vi "Generate Doku Syntax.vi"(5 "GitHub Base Path":string="https://github.com/labviewhacker/LVH-Toolbox/raw/master/LabVIEW/vi.lib/LabVIEW%20Hacker/LVH-Toolbox/Common/Public/", 7 "Image Base Path":string="lib/exe/fetch.php?media=wiki:playground:dokugen:", 8 "Error In":errorcluster, 10 "VIs":T1[](array[typedef]), 11 "Doc Config":T2) -> (0 "Error Out":errorcluster)   [LabVIEW 2014, in "LMH-Toolbox.lvlib" / "LMH-Documentation.lvlib"]
uses:
  <vilib>/MakerHub/Toolbox/Private/Documentation/LMH-Documentation.lvlib
  <vilib>/MakerHub/Toolbox/Private/Documentation/Private/Type Defs/Doc Config.ctl
  <vilib>/MakerHub/Toolbox/Private/Documentation/Private/Type Defs/VI.ctl
panel:
  out "array of strings 2":string[][](array[string])
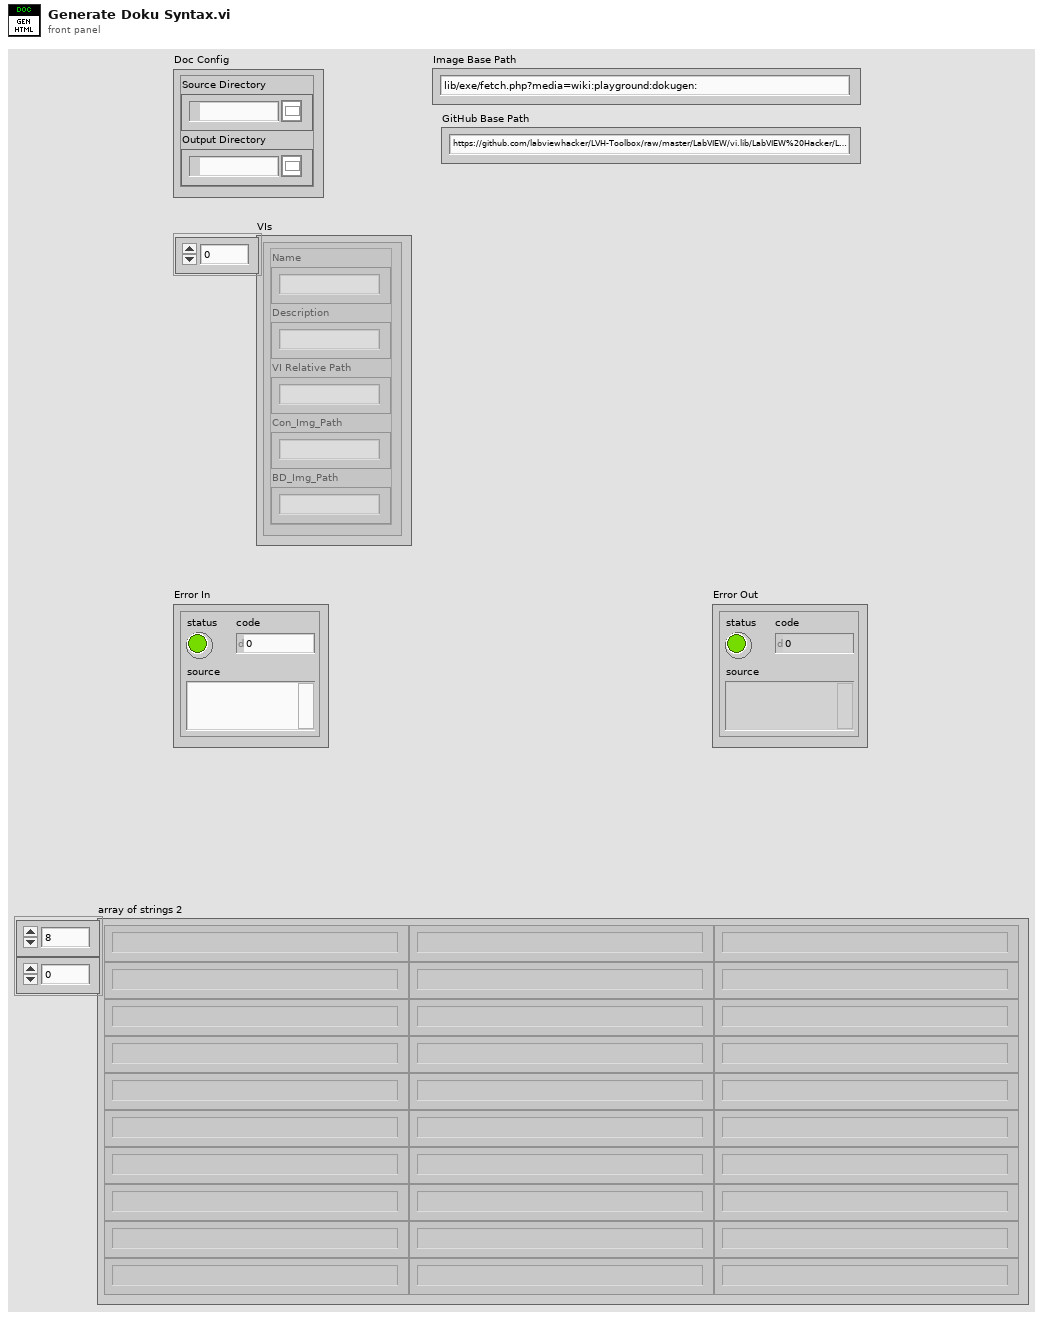
[diagram p1: front panel]
types:
  T1 = typedef "LMH-Toolbox.lvlib/LMH-Documentation.lvlib/VI.ctl" = cluster{"Name":string, "Description":string, "VI Relative Path":string, "Con_Img_Path":string, "BD_Img_Path":string}
  T2 = typedef "LMH-Toolbox.lvlib/LMH-Documentation.lvlib/Doc Config.ctl" = cluster{"Source Directory":path, "Output Directory":path}
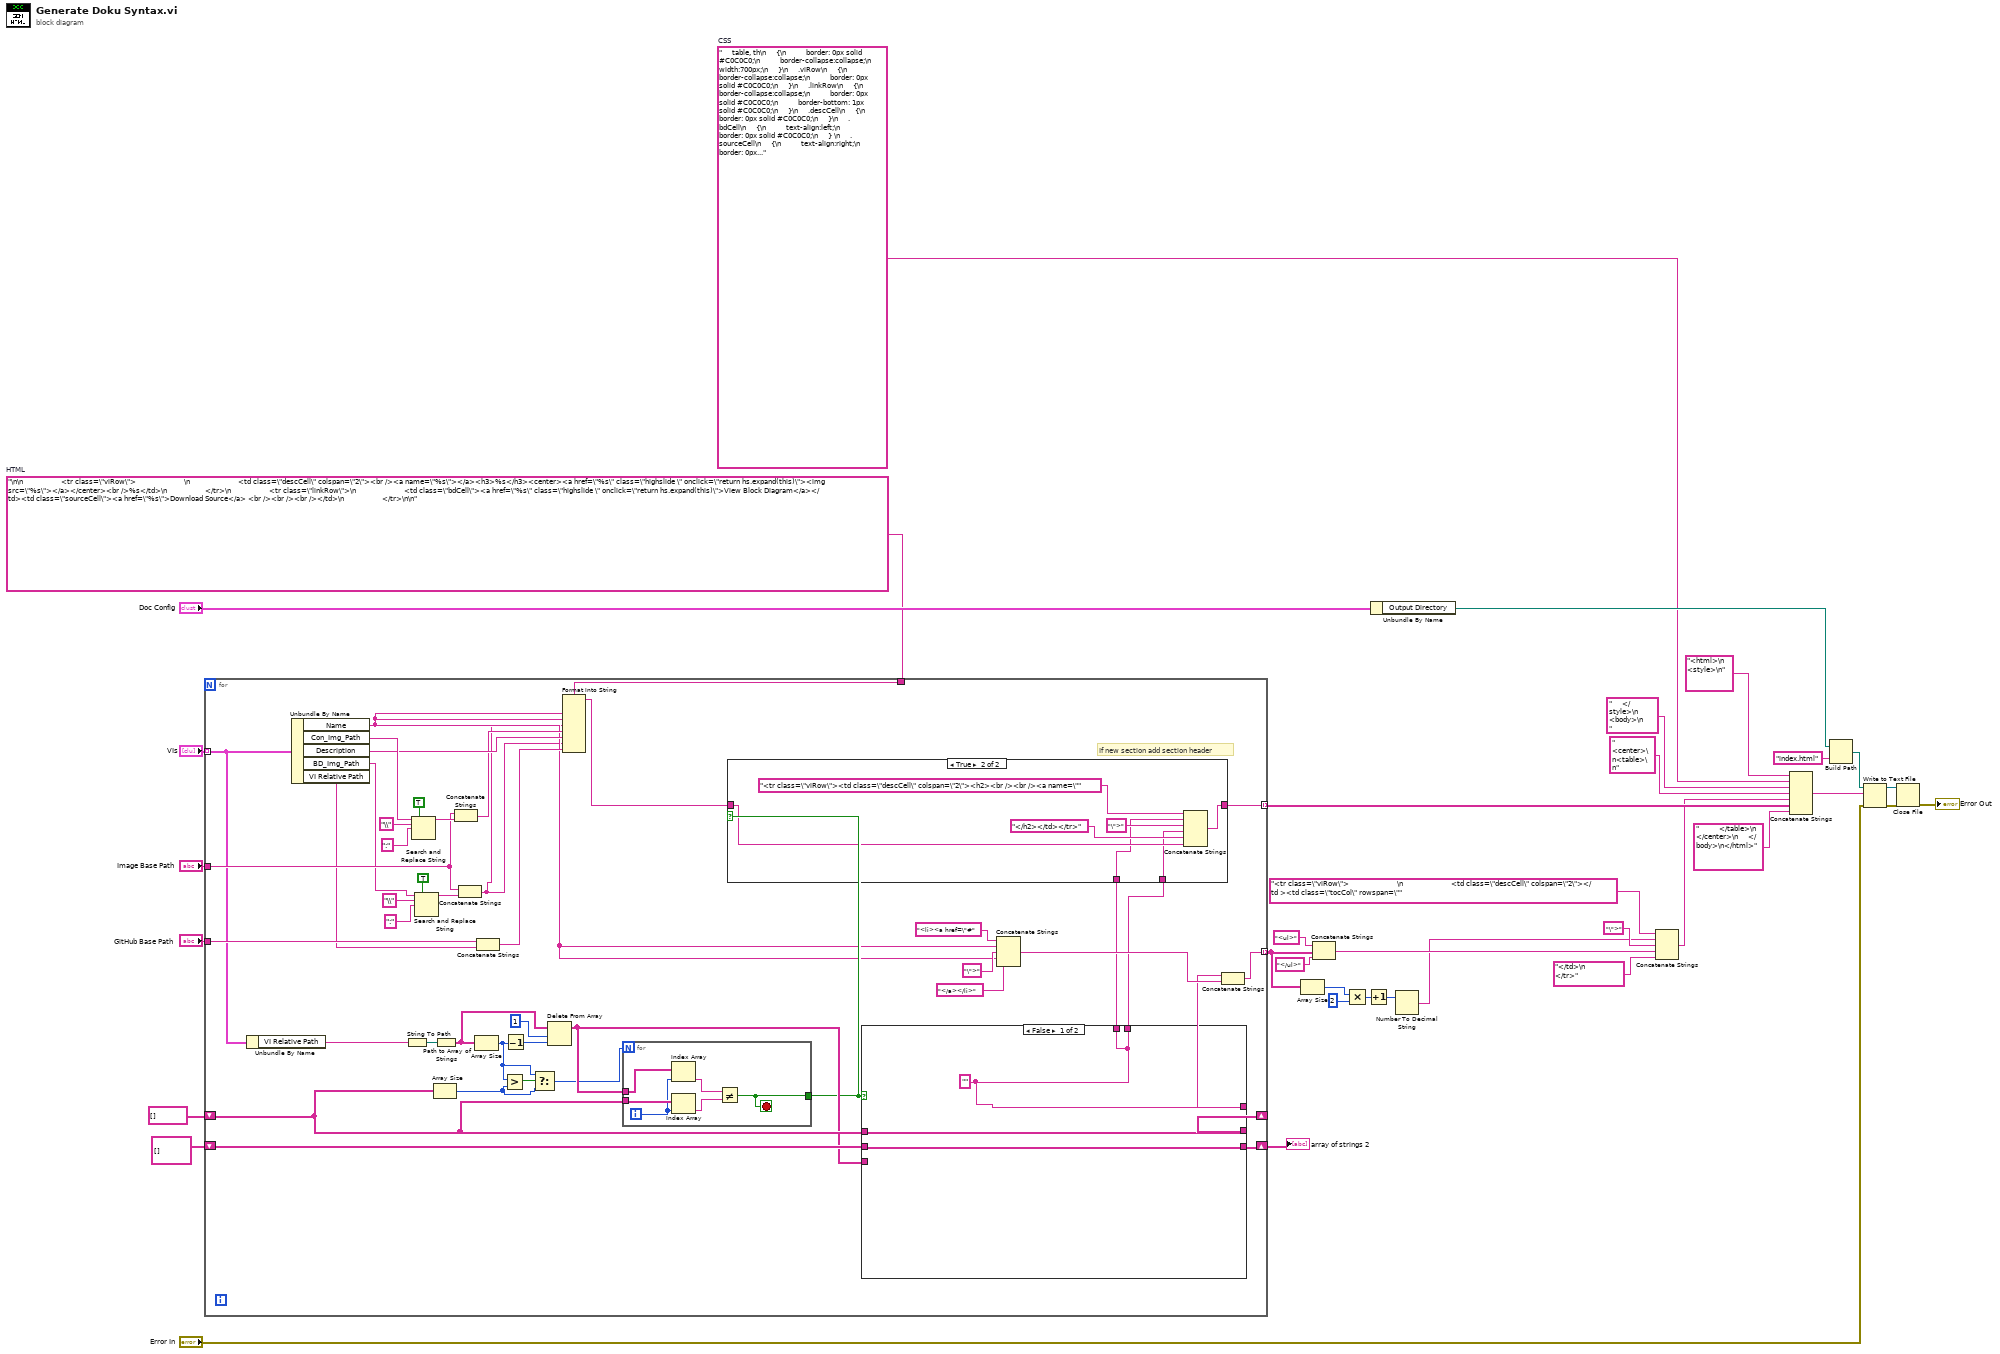
[diagram p0: block diagram]
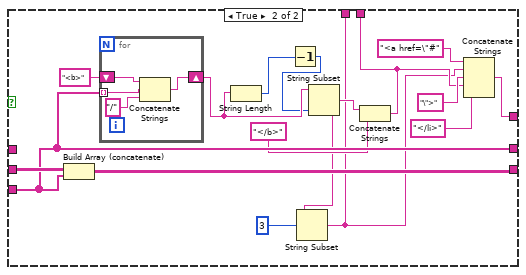
[diagram p3: hidden frame]
diagram:
  w20 = "\n\n                   <tr class=\"viRow\">                        \n                        <td class=\"descCell\" colspan=\"2\"><br /><a name=\"%s\"></a><h3>%s</h3><center><a href=\"%s\" class=\"highslide \" onclick=\"return hs.expand(this)\"><img src=\"%s\"></a></center><br />%s</td>\n                   </tr>\n                   <tr class=\"linkRow\">\n                        <td class=\"bdCell\"><a href=\"%s\" class=\"highslide \" onclick=\"return hs.expand(this)\">View Block Diagram</a></td><td class=\"sourceCell\"><a href=\"%s\">Download Source</a> <br /><br /><br /></td>\n                   </tr>\n\n"  # HTML
  w23 = "     table, th\n     {\n          border: 0px solid #C0C0C0;\n          border-collapse:collapse;\n          width:700px;\n     }\n     .viRow\n     {\n          border-collapse:collapse;\n          border: 0px solid #C0C0C0;\n     }\n     .linkRow\n     {\n          border-collapse:collapse;\n          border: 0px solid #C0C0C0;\n          border-bottom: 1px solid #C0C0C0;\n     }\n     .descCell\n     {\n           border: 0px solid #C0C0C0;\n     }\n     .bdCell\n     {\n          text-align:left;\n         border: 0px solid #C0C0C0;\n     } \n     .sourceCell\n     {\n          text-align:right;\n          border: 0px solid #C0C0C0;\n     } \n     .tocCol\n     {\n          border: 0px solid #C0C0C0;\n          width:300px;\n     } \n"  # CSS
  n1 = for {
    tunnel: "VIs" -> [w61] mode=indexing
    tunnel: "GitHub Base Path" -> [w64]
    tunnel: "Image Base Path" -> [w65]
    tunnel: w20 -> [w76]
    tunnel: [w43] -> w18 mode=indexing
    tunnel: [w45] -> w11 mode=indexing
    shift-right: [w57] -> _
    shift-left: string[] [] ("y") -> [w60]
    shift-right: [w58] -> w1
    shift-left: string[][] [] ("array of strings") -> [w59]
    # "If new section add section header"
    n2 = Unbundle By Name(w61) -> ("VI Relative Path"=w55:string)
    n3 = Unbundle By Name(w61) -> ("Name"=w41:string, "Con_Img_Path"=w77:string, "Description"=w75:string, "BD_Img_Path"=w40:string, "VI Relative Path"=w63:string)
    n4 = String To Path(string=w55) -> (path=w54:path)
    n5 = Search and Replace String(replace all?=TRUE ("replace all? (F)"), input string=w77, search string="\\", replace string=":" ("replace string (\"\")")) -> (result string=w74:string)  [unwired: 4 in, 3 out]
    n6 = Search and Replace String(replace all?=TRUE ("replace all? (F)"), input string=w40, search string="\\", replace string=":" ("replace string (\"\")")) -> (result string=w69:string)  [unwired: 4 in, 3 out]
    n7 = Array Size(array=w60) -> (size(s)=w48:i32)
    n8 = Path to Array of Strings(0:w54) -> (2:w51:string[])  [unwired: 1 out]
    n9 = Concatenate Strings(w65, w74) -> (w73:string)
    n10 = Concatenate Strings(w65, w69) -> (w39:string)
    n11 = Array Size(array=w51) -> (size(s)=w49:i32)
    n12 = Concatenate Strings(w64, w63) -> (w62:string)
    n13 = Greater?(x=w49, y=w48) -> (0:w50:bool)
    n14 = Decrement(x=w49) -> (x-1=w53:i32)
    n15 = Select(t=w49, s=w50, f=w48) -> (s? t:f=w47:i32)
    n16 = Delete From Array(array=w51, length=1, index=w53) -> (array with subset deleted=w56:string[])  [unwired: 1 out]
    n17 = Format Into String(format string=w76, w41, w41, w39, w73, w75, w39, w62) -> (resulting string=w44:string)  [unwired: 2 in, 1 out]
    n18 = for {
      N: w47 -> [_]
      tunnel: w60 -> [w92]
      tunnel: w56 -> [w93]
      tunnel: [w94] -> w42
      i -> [w91]
      stop <- w94 stop-if-true
      n19 = Index Array(array=w93, index=w91) -> (element=w89:string)
      n20 = Index Array(array=w92, index=w91) -> (element=w90:string)
      n21 = Not Equal?(x=w89, y=w90) -> (x != y?=w94:bool)
    }
    n22 = case shown="False" w42 {
      tunnel: w59 -> [w97 w112]
      tunnel: [w97 w113] -> w58
      tunnel: w56 -> [_ w111]
      tunnel: [w96 w111] -> w57
      tunnel: w60 -> [w96 _]
      tunnel: [w95 w102] -> w38
      tunnel: [w95 w101] -> w37
      tunnel: [w95 w98] -> w36
      frame False {
        w95 = ""
      }
      frame True {
        n23 = Build Array (concatenate)(w112, w111) -> (w113:string[][])
        n24 = for {
          tunnel: w111 -> [w114] mode=indexing
          shift-right: [w116] -> w109
          shift-left: "<b>" -> [w115]
          n25 = Concatenate Strings(w115, w114, "/" ("element")) -> (w116:string)
        }
        n26 = String Length(string=w109) -> (length=w108:i32)
        n27 = Decrement(x=w108) -> (x-1=w107:i32)
        n28 = String Subset(string=w109, length (rest)=w107) -> (substring=w99:string)  [unwired: 1 in]
        n29 = String Subset(string=w99, offset (0)=3) -> (substring=w98:string)  [unwired: 1 in]
        n30 = Concatenate Strings(w99, "</b>") -> (w101:string)
        n31 = Concatenate Strings("<a href=\"#" ("string"), w98, "\">" ("string"), w101, "</li>" ("string")) -> (w102:string)
      }
    }
    n32 = case shown="True" w42 {
      tunnel: w44 -> [w81 w86]
      tunnel: [w81 w88] -> w43
      tunnel: w37 -> [_ w83]
      tunnel: w36 -> [_ w82]
      frame False {
      }
      frame True {
        n33 = Concatenate Strings("<tr class=\"viRow\"><td class=\"descCell\" colspan=\"2\"><h2><br /><br /><a name=\"" ("string"), w82, "\">" ("string"), w83, "</h2></td></tr>" ("string"), w86) -> (w88:string)
      }
    }
    n34 = Concatenate Strings("<li><a href=\"#" ("string"), w41, "\">" ("string"), w41, "</a></li>" ("string")) -> (w46:string)
    n35 = Concatenate Strings(w38, w46) -> (w45:string)
  }
  "array of strings 2" <- w1
  n36 = Array Size(array=w11) -> (size(s)=w7:i32)
  n37 = Concatenate Strings("<ul>", w11, "</ul>" ("string")) -> (w14:string)
  n38 = Multiply(x=w7, y=2) -> (x*y=w5:i32)
  n39 = Increment(x=w5) -> (x+1=w4:i32)
  n40 = Unbundle By Name("Doc Config") -> ("Output Directory"=w32:path)
  n41 = Number To Decimal String(number=w4) -> (decimal integer string=w8:string)  [unwired: 1 in]
  n42 = Concatenate Strings("<tr class=\"viRow\">                        \n                        <td class=\"descCell\" colspan=\"2\"></td ><td class=\"tocCol\" rowspan=\"" ("string"), w8, "\">" ("string"), w14, "</td>\n                   </tr>" ("string")) -> (w12:string)
  n43 = Concatenate Strings("<html>\n     <style>\n", w23, "     </style>\n     <body>\n              " ("string"), " <center>\n<table>\n" ("string"), w12, w18, "          </table>\n          </center>\n     </body>\n</html>") -> (w34:string)
  n44 = Build Path(base path=w32, name or relative path="index.html") -> (appended path=w30:path)
  n45 = Write to Text File(file (use dialog)=w30, text=w34, error in="Error In") -> (refnum out=w28:refnum<file>, error out=w29:errorcluster)  [unwired: 1 in, 1 out]
  n46 = Close File(refnum=w28, error in=w29) -> (error out=→"Error Out":errorcluster)  [unwired: 1 out]
